vi "Mexa D RT.vi"() -> ()   [LabVIEW 2011]
uses:
  <vilib>/rvi/interface/nirviOpenFPGA/nirviOpenFPGA.xnode
  <vilib>/rvi/interface/nirviReadWriteControl/nirviReadWriteControl.xnode
  <vilib>/rvi/interface/Simulation/niFpgaSimulationCallBeginRW.vi
  <vilib>/rvi/errors/niLvFpgaAdjustHostInterfaceError.vi
  <vilib>/rvi/interface/nirviCloseFPGA/nirviCloseFPGA.xnode
  NiFpgaLv.dll
  <vilib>/Utility/error.llb/Error Cluster From Error Code.vi
  <vilib>/FPGAPlugInAG/Dynamic/niLvFpga_Close_Dynamic.vi
  Mexa MAX FPGA D.vi
panel:
  in  "stop":bool
  in  "Turn Off Measurement":bool
  in  "Turn On Measurement":bool
  out "Output":dbl[](array[numeric])
  # "CO2 %"
  # "CO %"
  # "HC ppm"
  # "O2 %"
  # "NOx ppm"
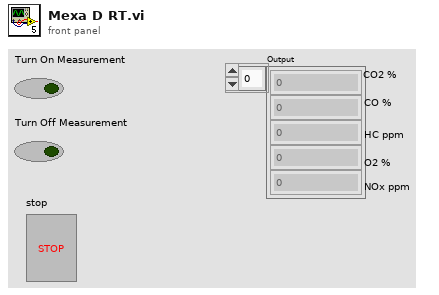
[diagram p1: front panel]
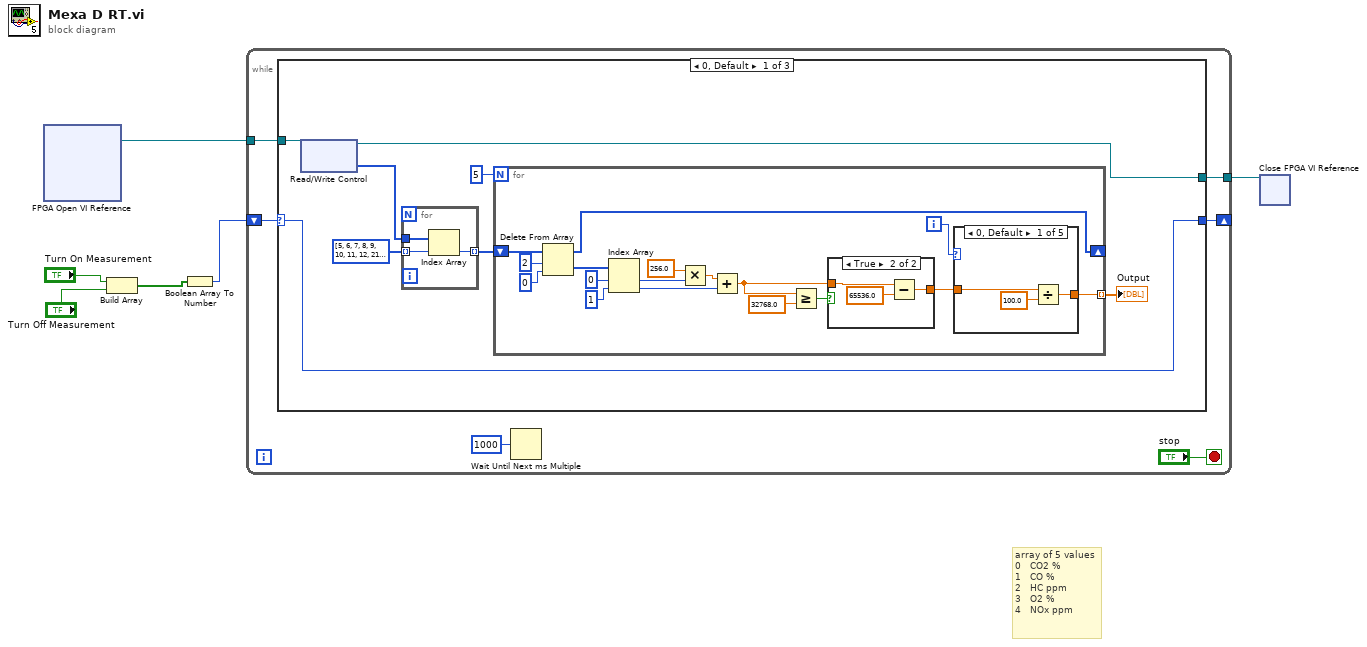
[diagram p0: block diagram]
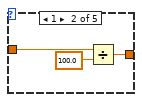
[diagram p2: hidden frame]
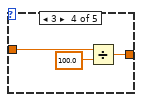
[diagram p4: hidden frame]
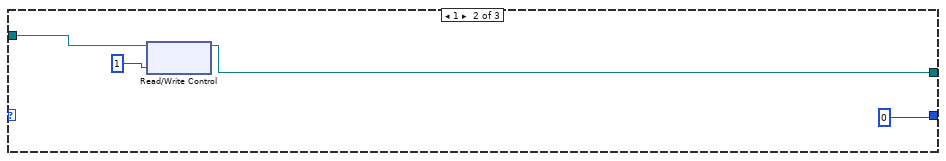
[diagram p7: hidden frame]
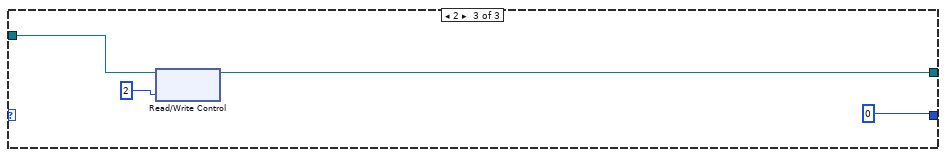
[diagram p8: hidden frame]
diagram:
  # "array of 5 values\n0   CO2 %\n1   CO %\n2   HC ppm\n3   O2 %\n4   NOx ppm"
  n1 = xnode "FPGA Open VI Reference"() -> ("FPGA VI Reference Out"=w2:refnum<k20>)  [unwired: 2 in, 1 out]
  n2 = Build Array("Turn On Measurement", "Turn Off Measurement") -> (w4:bool[])
  n3 = Boolean Array To Number(Boolean array=w4) -> (number=w3:u32)
  n4 = while {
    tunnel: w2 -> [w11]
    shift-right: [w10] -> _
    shift-left: w3 -> [w12]
    tunnel: [w8] -> w1
    stop <- "stop" stop-if-true
    n5 = case shown="0, Default" w12 {
      selector: w12 -> [w14 _ _]
      tunnel: w11 -> [w20 w58 w62]
      tunnel: [w14 i16 0 ("Numeric") i16 0 ("Numeric")] -> w10
      tunnel: [w13 w56 w60] -> w8
      frame 0, Default {
        n6 = xnode "Read/Write Control"("FPGA VI Reference In"=w20) -> ("FPGA VI Reference Out"=w13:refnum<k20>, "Output"=w15:u8[])  [unwired: 1 in, 1 out]
        n7 = for {
          tunnel: w15 -> [w55]
          tunnel: i32[] [5, 6, 7, 8, 9, 10, 11, 12, 21, 22] -> [w54] mode=indexing
          tunnel: [w53] -> w17 mode=indexing
          n8 = Index Array(array=w55, index=w54) -> (element=w53:u8)
        }
        n9 = for {
          N: 5 -> [_]
          shift-right: [w31] -> _
          shift-left: w17 -> [w37]
          tunnel: [w21] -> w19 mode=indexing
          i -> [w23]
          n10 = Delete From Array(array=w37, length=2, index=0) -> (deleted portion=w34:u8[], array with subset deleted=w31:u8[])
          n11 = Index Array(array=w34, index #1=0 ("index"), index #2=1 ("index")) -> (element #1=w29:u8, element #2=w27:u8)
          n12 = Multiply(x=256.0, y=w29) -> (x*y=w28:dbl)
          n13 = Add(x=w28, y=w27) -> (x+y=w24:dbl)
          n14 = Greater Or Equal?(x=w24, y=32768.0) -> (x >= y?=w26:bool)
          n15 = case shown="True" w26 {
            tunnel: w24 -> [w49 w52]
            tunnel: [w49 w51] -> w22
            frame False {
            }
            frame True {
              n16 = Subtract(x=w52, y=65536.0) -> (x-y=w51:dbl)
            }
          }
          n17 = case shown="0, Default" w23 {
            tunnel: w22 -> [w40 w41 w44 w45 w48]
            tunnel: [w38 w42 w44 w46 w48] -> w21
            frame 0, Default {
              n18 = Divide(x=w40, y=100.0) -> (x/y=w38:dbl)
            }
            frame 1 {
              n19 = Divide(x=w41, y=100.0) -> (x/y=w42:dbl)
            }
            frame 2 {
            }
            frame 3 {
              n20 = Divide(x=w45, y=100.0) -> (x/y=w46:dbl)
            }
            frame 4 {
            }
          }
        }
        "Output" <- w19
      }
      frame 1 {
        n21 = xnode "Read/Write Control"("FPGA VI Reference In"=w58, "Numeric"=i16 1) -> ("FPGA VI Reference Out"=w56:refnum<k20>)  [unwired: 1 in, 1 out]
      }
      frame 2 {
        n22 = xnode "Read/Write Control"("FPGA VI Reference In"=w62, "Numeric"=i16 2) -> ("FPGA VI Reference Out"=w60:refnum<k20>)  [unwired: 1 in, 1 out]
      }
    }
    n23 = Wait Until Next ms Multiple(millisecond multiple=u32 1000) -> ()  [unwired: 1 out]
  }
  n24 = xnode "Close FPGA VI Reference"("FPGA VI Reference In"=w1) -> ()  [unwired: 1 in, 1 out]
